vi "FTW-Scripter-Core_OnLoadScript.vi"(0 "FTW-Scripter-Core In":refnum<class "FTW-Scripter-Core.lvclass">, 5 "Script":string, 11 "error in":errorcluster) -> (4 "FTW-Scripter-Core Out":refnum<class "FTW-Scripter-Core.lvclass">, 15 "error out":errorcluster)   [LabVIEW 2015, in "FTW-Scripter-Core.lvclass"]
uses:
  FTW-Scripter-Core.lvclass
  FTW-Scripter_Step.ctl
  FTW-Scripter-Core.lvclass/FTW-Scripter-Core.ctl
  source/container/FTW-Container.lvclass
panel:
  out "Loaded Script":T1[](array[typedef])
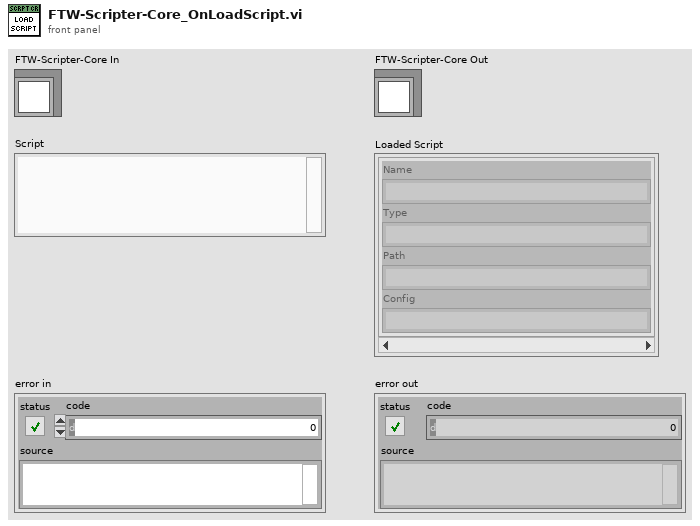
[diagram p1: front panel]
types:
  T1 = typedef "FTW-Scripter_Step.ctl" = cluster{"Name":string, "Type":string, "Path":string, "Config":string}
  T2 = enum8{"Unloaded", "Loaded", "Executing", "Paused"}
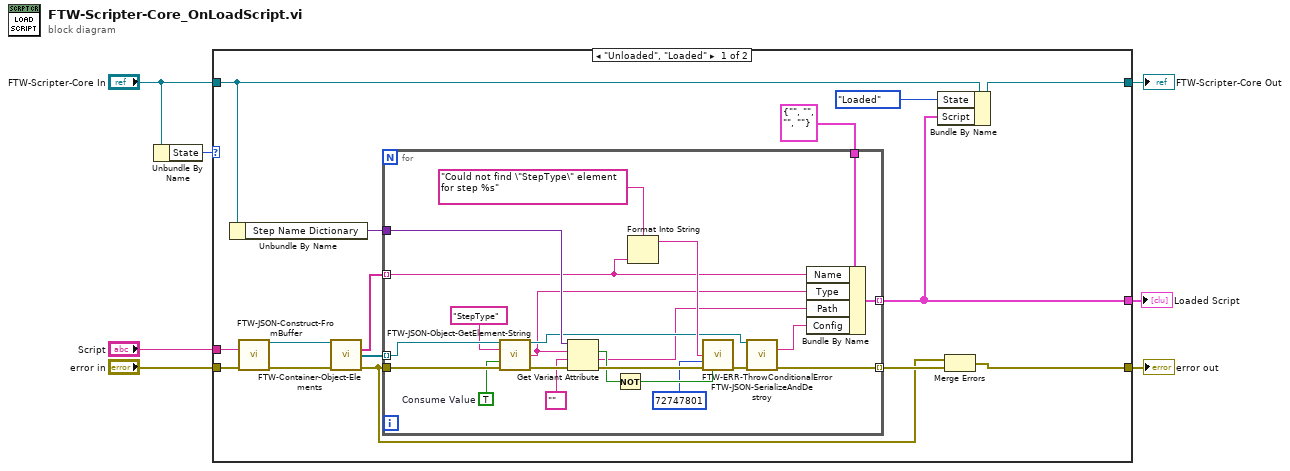
[diagram p0: block diagram]
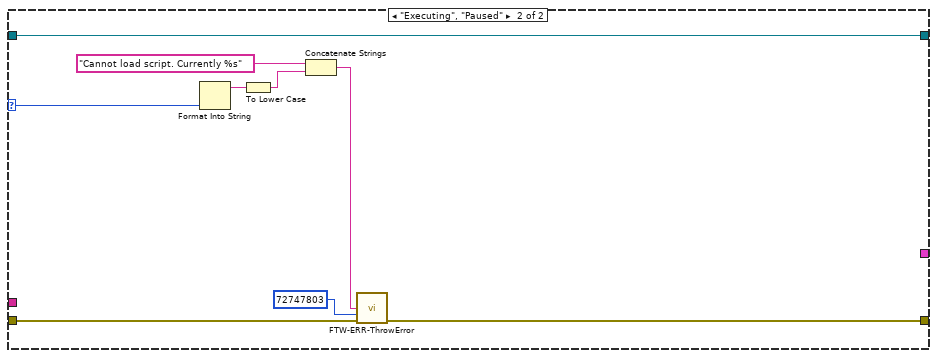
[diagram p2: hidden frame]
diagram:
  n1 = Unbundle By Name("FTW-Scripter-Core In") -> ("State"=w5:T2)
  n2 = case shown="\"Unloaded\", \"Loaded\"" w5 {
    selector: w5 -> [_ w49]
    tunnel: [w21 w53] -> w7
    tunnel: "FTW-Scripter-Core In" -> [w10 w53]
    tunnel: [w12 w51] -> w4
    tunnel: "error in" -> [w22 w52]
    tunnel: "Script" -> [w18 _]
    tunnel: [w8 _] -> w1
    frame "Unloaded", "Loaded" {
      n3 = Unbundle By Name(w10) -> ("Step Name Dictionary"=w15:variant)
      n4 = call "FTW-JSON-Construct-FromBuffer.vi"("JSON String (UTF-8)"=w18, "error in"=w22) -> ("JSON"=w17:refnum<class "FTW-Container.lvclass">, "error out"=w19:errorcluster)  [unwired: 12 in]
      n5 = call "FTW-Container-Object-Elements.vi"("FTW-Container In"=w17, "error in"=w19) -> ("Names"=w20:string[], "Object Elements"=w16:refnum<class "FTW-Container.lvclass">[], "error out"=w11:errorcluster)  [unwired: 10 in, 1 out]
      n6 = for {
        tunnel: w20 -> [w28] mode=indexing
        tunnel: w11 -> [w43]
        tunnel: w16 -> [w44] mode=indexing
        tunnel: w15 -> [w38]
        tunnel: [w30] -> w13 mode=indexing
        tunnel: [w27] -> w8 mode=indexing
        tunnel: T1 {"Name"="", "Type"="", "Path"="", "Config"=""} ("element") -> [w23]
        w41 = TRUE  # Consume Value
        n7 = call "FTW-JSON-Object-GetElement-String.vi"("JSON"=w44, "Key"="StepType", "Consume Value"=w41, "error in"=w43) -> ("JSON out"=w29:refnum<class "FTW-Container.lvclass">, "Value"=w25:string, "error out"=w40:errorcluster)  [unwired: 7 in, 2 out]
        n8 = Get Variant Attribute(Variant=w38, name=w25, default value (empty Variant)="" ("empty string"), error in=w40) -> (found=w35:bool, value=w24:string, error out=w37:errorcluster)  [unwired: 1 out]
        n9 = Not(x=w35) -> (.not. x?=w34:bool)
        n10 = Format Into String(format string="Could not find \"StepType\" element for step %s" ("Error Message"), w28) -> (resulting string=w32:string)  [unwired: 2 in, 1 out]
        n11 = call "FTW-ERR-ThrowConditionalError.vi"("Error Message"=w32, "Error Code"=72747801, "error in"=w37, "Throw Error?"=w34) -> ("error out"=w36:errorcluster)  [unwired: 11 in]
        n12 = call "FTW-JSON-SerializeAndDestroy.vi"("JSON"=w29, "error in"=w36) -> ("JSON String (UTF-8)"=w26:string, "error out"=w30:errorcluster)  [unwired: 12 in]
        n13 = Bundle By Name(cluster=w23, "Name"=w28, "Type"=w25, "Path"=w24, "Config"=w26) -> (w27:T1)
      }
      n14 = Bundle By Name(cluster=w10, "State"=T2."Loaded", "Script"=w8) -> (w21:refnum<class "FTW-Scripter-Core.lvclass">)
      n15 = Merge Errors(w11, w13) -> (w12:errorcluster)
    }
    frame "Executing", "Paused" {
      n16 = Format Into String(w49) -> (resulting string=w48:string)  [unwired: 3 in, 1 out]
      n17 = To Lower Case(string=w48) -> (all lower case string=w46:string)
      n18 = Concatenate Strings("Cannot load script. Currently %s" ("Error Message"), w46) -> (w47:string)
      n19 = call "FTW-ERR-ThrowError.vi"("Error Message"=w47, "Error Code"=72747803, "error in"=w52) -> ("error out"=w51:errorcluster)  [unwired: 12 in]
    }
  }
  "FTW-Scripter-Core Out" <- w7
  "error out" <- w4
  "Loaded Script" <- w1
